vi "Replace with Magnitude.vi"(11 "String In":string) -> (3 "String Out":string)   [LabVIEW 2021]
uses:
  <vilib>/regexp/Match Regular Expression.xnode
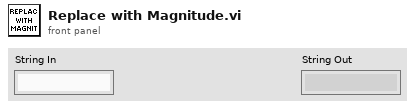
[diagram p1: front panel]
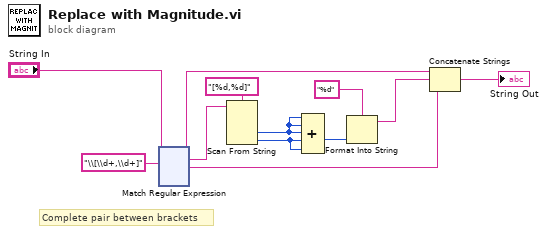
[diagram p0: block diagram]
diagram:
  # "Complete pair between brackets"
  n1 = xnode "Match Regular Expression"("input string"="String In", "regular expression"="\\[\\d+,\\d+]") -> ("before match"=w8:string, "whole match"=w7:string, "after match"=w10:string)  [unwired: 4 in, 2 out]
  n2 = Scan From String(format string="[%d,%d]" ("regular expression"), input string=w7) -> (output 1=w5:i32, output 2=w4:i32)  [unwired: 4 in, 3 out]
  n3 = Compound Arithmetic op=ADD(w5, w5, w5, w4, w4) -> (w3:i32)
  n4 = Format Into String(format string="%d", w3) -> (resulting string=w1:string)  [unwired: 2 in, 1 out]
  n5 = Concatenate Strings(w8, w1, w10) -> (→"String Out":string)
